vi "Demo Dialog.vi"(8 "error in (no error)":errorcluster) -> (0 "error out":errorcluster)   [LabVIEW 2011]
uses:
  VIremote.llb/VIremoteEvent.ctl
  VIremote.llb/VIremoteFunction.ctl
  <vilib>/Utility/error.llb/DialogType.ctl
panel:
  in  "Error dialog":bool
  in  "Alert":bool
  in  "Title":string="Dialog test"
  out "Button tap:":string
  in  "Buttons":T1={"Button 0"="Button 0", "Button 1"="Button 1", "Button 2"="Button number two"}
  in  "Dialog":bool
  in  "VIremoteEvent":T2=enum."Connection Closed"
  in  "Message":string="My test message"
  # "Tap the left button below to bring up a Button Dialog with the above info. The VIremoteButtonDialog.vi will return with the button index when a button is clicked. You can have more than three buttons if you need (or less). The \"Show Alert message\" function will return immediately (not waiting for the OK button)."
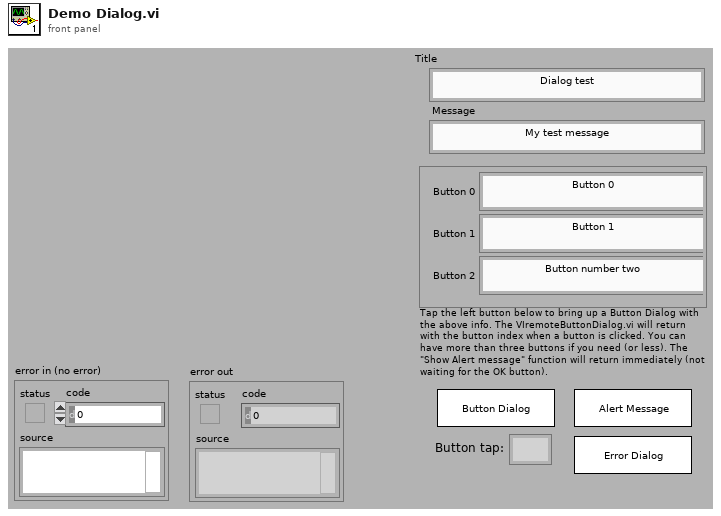
[diagram p1: front panel]
types:
  T1 = cluster{"Button 0":string, "Button 1":string, "Button 2":string}
  T2 = typedef "VIremoteEvent.ctl" = enum16{"No Event", "Connection Closed", "Navigate Back", "Enter Background", "Enter Foreground", "Portrait", "Portrait Upside Down", "Landscape Left", "Landscape Right"}
  T3 = typedef "VIremoteFunction.ctl" = enum16{"Do nothing", "Stop controller", "Close this connection", "Show info panel", "Set VI to control", "Set Accelerometer freq (Hz)", "Show Alert message", "Start Sound Input", "Stop Sound Input", "Set Volume (0-100)", "Set sound output Speaker", "Set sound output Receiver", "Play Sound", "Repeat Sound", "Stop Sound", "Pause Sound", "Resume Sound", "Set panel width of caller (320 or 480)", "Set Panel Size to Portrait", "Set Panel Size to Landscape", "Set Panel Size as Current Orientation", "Allow all UI Orientations", "Send user notification", "Disable Scrolling", "Normal Scrolling", "Page Scrolling", "Set Scroll Offset", "Page Indicator Position"}
  T4 = typedef "DialogType.ctl" = u16
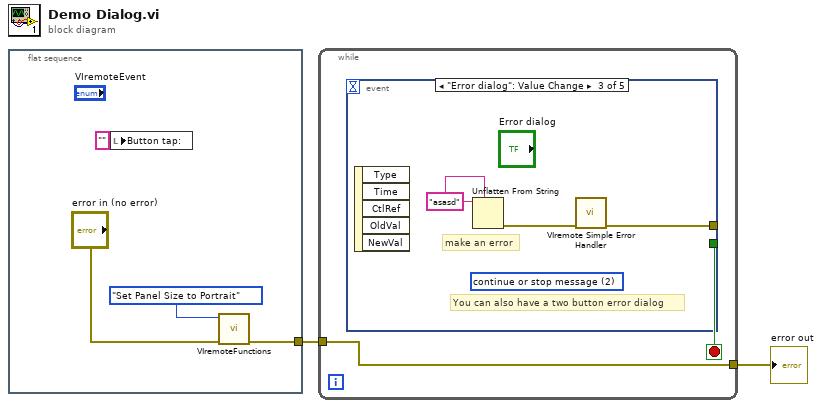
[diagram p0: block diagram]
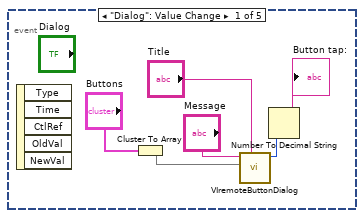
[diagram p2: hidden frame]
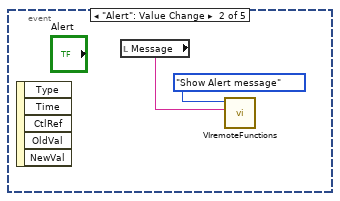
[diagram p3: hidden frame]
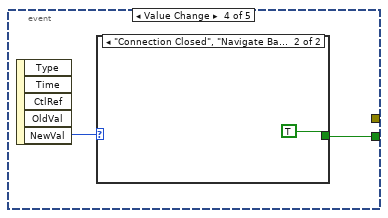
[diagram p4: hidden frame]
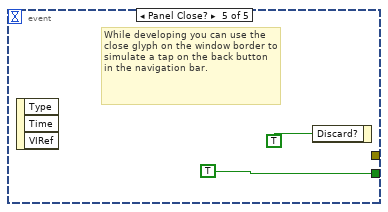
[diagram p6: hidden frame]
diagram:
  n1 = flat-sequence {
    tunnel: [w5] -> w2
    frame #0 {
      n2 = local write "Button tap:"("" ("Button tap:")) -> ()
      n3 = call "VIremoteFunctions.vi"("error in (no error)"="error in (no error)", "Function"=VIremoteFunction."Set Panel Size to Portrait") -> ("error out"=w5:errorcluster)  [unwired: 4 in, 5 out]
    }
  }
  n4 = while {
    tunnel: w2 -> [w7]
    tunnel: [w7] -> w1
    stop <- w8 stop-if-true
    n5 = event shown="[2] \"Error dialog\": Value Change" {
      selector: _ -> [_ _ _ _ _]
      dyn-events: _ -> [_ _ _ _ _]
      timeout: _ -> [_ _ _ _ _]
      tunnel: [_ _ _ w20 TRUE ("Discard?")] -> w8
      tunnel: [_ _ w17 _ _] -> _
      event "Dialog": Value Change {
        n6 = event-data() -> ()  [unwired: 6 out]
        n7 = Cluster To Array(cluster="Buttons") -> (array=w13:string[])
        n8 = call "VIremoteButtonDialog.vi"("Window Title (\"\")"="Title", "Buttons(OK)"=w13, "message"="Message") -> ("Which Button? (-1 if connection lost)"=w12:i32)  [unwired: 1 in, 7 out]
        n9 = Number To Decimal String(number=w12) -> (decimal integer string=→"Button tap:":string)  [unwired: 1 out]
      }
      event "Alert": Value Change {
        n10 = event-data() -> ()  [unwired: 6 out]
        n11 = local read "Message"() -> (w15:string)
        n12 = call "VIremoteFunctions.vi"("String in"=w15, "Function"=VIremoteFunction."Show Alert message") -> ()  [unwired: 4 in, 6 out]
      }
      event "Error dialog": Value Change {
        (unwired) T4 2 items=["no dialog", "OK message", "continue or stop message", "OK message + warnings", "continue/stop + warnings"] ("type of dialog (OK msg:1)")
        w19 = "asasd" ("binary string")
        # "You can also have a two button error dialog"
        # "make an error"
        n13 = event-data() -> ()  [unwired: 6 out]
        n14 = Unflatten From String(type=w19, binary string=w19) -> (error out=w18:errorcluster)  [unwired: 1 in, 4 out]
        n15 = call "VIremote Simple Error Handler.vi"("error in (no error)"=w18) -> ("error out"=w17:errorcluster)  [unwired: 1 in, 7 out]
      }
      event Value Change {
        n16 = event-data() -> ("NewVal"=w21:T2)  [unwired: 5 out]
        n17 = case shown="\"Connection Closed\", \"Navigate Back\"" w21 {
          tunnel: [_ TRUE] -> w20
          frame "No Event", Default {
          }
          frame "Connection Closed", "Navigate Back" {
          }
        }
      }
      event Panel Close? {
        # "While developing you can use the close glyph on the window border to simulate a tap on the back button in the navigation bar."
        n18 = event-data() -> ()  [unwired: 4 out]
        n19 = event-data("Discard?"=TRUE) -> ()  [unwired: 1 in, 1 out]
      }
    }
  }
  "error out" <- w1
